vi "Climb Command Handler Test.vi"(6 "Operator POVs":i16[](array[numeric]), 7 "Driver POVs":i16[](array[numeric]), 8 "Operator Axes":dbl[](array[numeric]), 9 "Operator Buttons":bool[](array[boolean]), 10 "Driver Buttons":bool[](array[boolean]), 11 "Driver Axes":dbl[](array[numeric])) -> ()   [LabVIEW 2019]
uses:
  Implementation/Climb Operations.ctl
  1425ab26-42c7-45e9-9c20-83b7d7a8b8c5.vi
panel:
  in  "Up":dbl
  in  "Down":dbl
  in  "Disengage":dbl
  in  "Engage":dbl
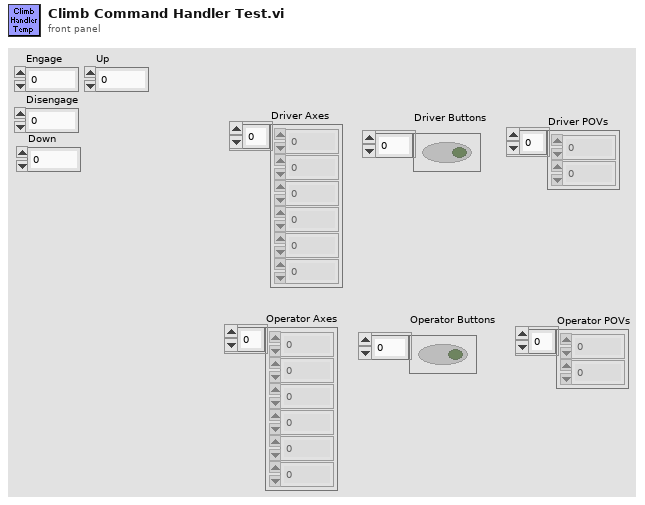
[diagram p1: front panel]
types:
  T1 = typedef "Climb Operations.ctl" = enum16{"Reserve", "Read Current", "Immediate Winch", "Immediate Servo"}
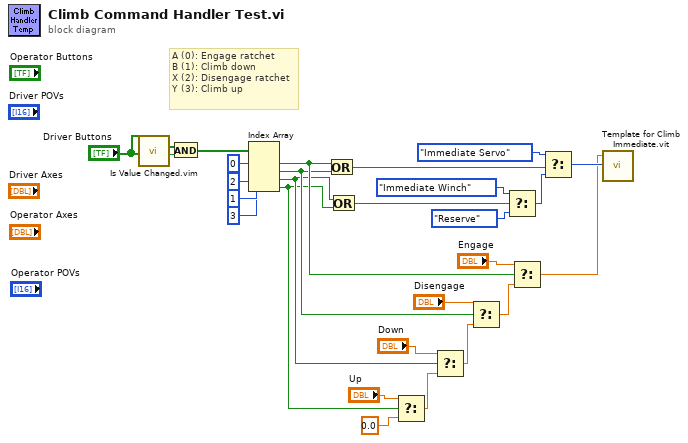
[diagram p0: block diagram]
diagram:
  # "A (0): Engage ratchet\nB (1): Climb down\nX (2): Disengage ratchet\nY (3): Climb up"
  n1 = call "Is Value Changed.vim"("value"="Driver Buttons") -> ("changed or first call?"=w1:bool)
  n2 = And(x="Driver Buttons", y=w1) -> (x .and. y?=w2:bool[])
  n3 = Index Array(array=w2, index #1=0 ("index"), index #2=2 ("index"), index #3=1 ("index"), index #4=3 ("index")) -> (element #1=w16:bool, element #2=w13:bool, element #3=w10:bool, element #4=w6:bool)
  n4 = Or(x=w16, y=w13) -> (x .or. y?=w18:bool)
  n5 = Or(x=w10, y=w6) -> (x .or. y?=w17:bool)
  n6 = Select(t="Up", s=w6, f=0.0) -> (s? t:f=w8:dbl)
  n7 = Select(t="Down", s=w10, f=w8) -> (s? t:f=w11:dbl)
  n8 = Select(t="Disengage", s=w13, f=w11) -> (s? t:f=w14:dbl)
  n9 = Select(t=Climb_Operations."Immediate Winch" ("Operation"), s=w17, f=Climb_Operations."Reserve" ("Operation")) -> (s? t:f=w20:T1)
  n10 = Select(t="Engage", s=w16, f=w14) -> (s? t:f=w4:dbl)
  n11 = Select(t=Climb_Operations."Immediate Servo" ("Operation"), s=w18, f=w20) -> (s? t:f=w22:T1)
  n12 = call "Template for Climb Immediate.vit"("Operation"=w22, "Setpoint"=w4) -> ()  [unwired: 9 in, 1 out]
